vi "콜라자판기(상태머신).vi"() -> ()   [LabVIEW 2014]
uses:
  Status.ctl
panel:
  out "Count Up":i32
  out "그림 링":u16(ring)
  in  "종료":bool
  in  "반환":bool
  in  "구매":bool
  out "투입금액":i32 format="%.0f원"
  in  "동전":T1
  # "콜라자판기"
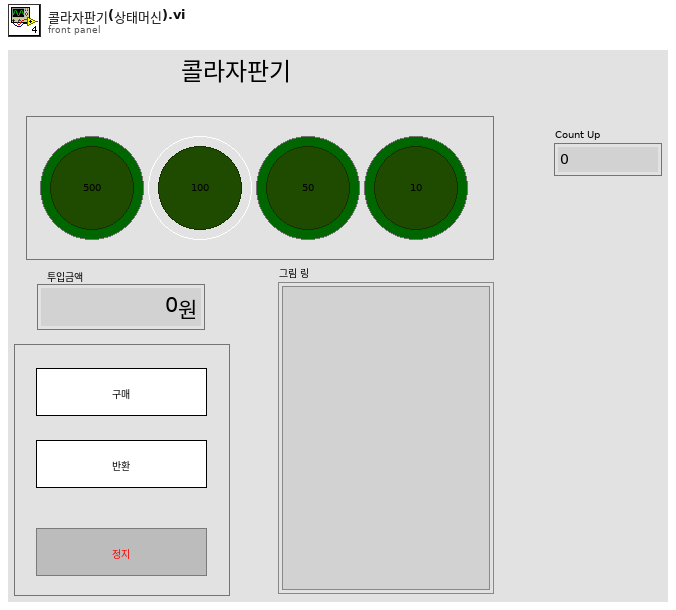
[diagram p1: front panel]
types:
  T1 = cluster{"불리언":bool, "불리언 2":bool, "불리언 3":bool, "불리언 4":bool}
  T2 = typedef "Status.ctl" = enum16{"Idle", "초기화", "종료", "구매", "반환", "1초기다림"}
  T3 = enum8{"Enabled", "Disabled", "Disabled and Grayed Out"}
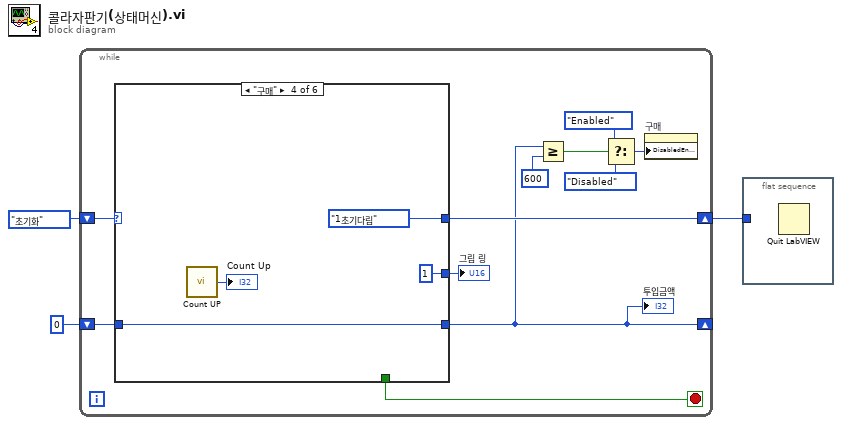
[diagram p0: block diagram]
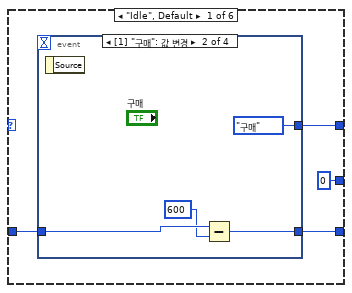
[diagram p2: hidden frame]
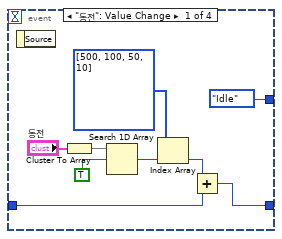
[diagram p3: hidden frame]
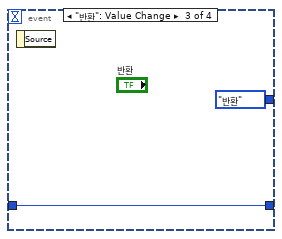
[diagram p4: hidden frame]
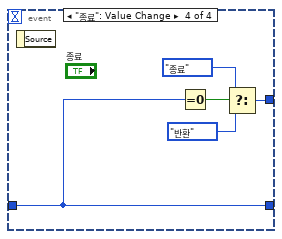
[diagram p5: hidden frame]
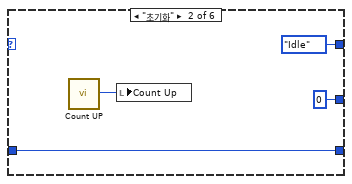
[diagram p6: hidden frame]
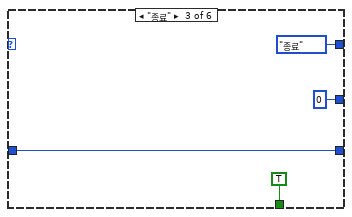
[diagram p7: hidden frame]
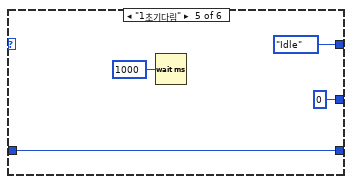
[diagram p8: hidden frame]
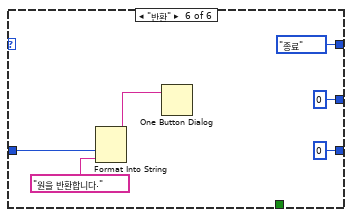
[diagram p9: hidden frame]
diagram:
  n1 = while {
    shift-right: [w13] -> w1
    shift-left: Status."초기화" ("Status") -> [w14]
    shift-right: [w5] -> _
    shift-left: 0 -> [w12]
    stop <- w6 stop-if-true
    n2 = case shown="\"구매\"" w14 {
      tunnel: [w18 Status."Idle" ("Status") Status."종료" ("Status") Status."1초기다림" ("Status") Status."Idle" ("Status") Status."종료" ("Status")] -> w13
      tunnel: w12 -> [w17 w40 w44 w49 w52 w60]
      tunnel: [w16 w40 w44 w49 w52 0] -> w5
      tunnel: [u16 0 u16 0 u16 0 u16 1 u16 0 u16 0] -> w4
      tunnel: [_ _ TRUE _ _ _] -> w6
      frame "Idle", Default {
        n3 = event shown="[1] \"구매\": 값 변경" {
          selector: _ -> [_ _ _ _]
          dyn-events: _ -> [_ _ _ _]
          timeout: _ -> [_ _ _ _]
          tunnel: [Status."Idle" ("Status") Status."구매" ("Status") Status."반환" ("Status") w34] -> w18
          tunnel: w17 -> [w20 w30 w32 w37]
          tunnel: [w19 w29 w32 w37] -> w16
          event "동전": Value Change {
            n4 = event-data() -> ()  [unwired: 1 in, 1 out]
            n5 = Cluster To Array(cluster="동전") -> (array=w25:bool[])
            n6 = Search 1D Array(1D array=w25, element=TRUE) -> (index of element=w23:i32)  [unwired: 1 in]
            n7 = Index Array(array=i32[] [500, 100, 50, 10], index=w23) -> (element=w21:i32)
            n8 = Add(x=w21, y=w20) -> (x+y=w19:i32)
          }
          event "구매": Value Change {
            n9 = event-data() -> ()  [unwired: 1 in, 1 out]
            n10 = Subtract(x=w30, y=600) -> (x-y=w29:i32)
          }
          event "반환": Value Change {
            n11 = event-data() -> ()  [unwired: 1 in, 1 out]
          }
          event "종료": Value Change {
            n12 = event-data() -> ()  [unwired: 1 in, 1 out]
            n13 = Equal To 0?(x=w37) -> (x = 0?=w38:bool)
            n14 = Select(t=Status."종료" ("Status"), s=w38, f=Status."반환" ("Status")) -> (s? t:f=w34:T2)
          }
        }
      }
      frame "초기화" {
        n15 = call "Count UP.vi"() -> ("Count Up"=w39:i32)
        n16 = local write "Count Up"(w39) -> ()
      }
      frame "종료" {
      }
      frame "구매" {
        n17 = call "Count UP.vi"() -> ("Count Up"=→"Count Up":i32)
      }
      frame "1초기다림" {
        n18 = Wait (ms)(milliseconds to wait=u32 1000 ("대기 시간(ms)")) -> ()  [unwired: 1 out]
      }
      frame "반환" {
        n19 = Format Into String(w60, "원을 반환합니다.") -> (resulting string=w58:string)  [unwired: 3 in, 1 out]
        n20 = One Button Dialog(message=w58) -> ()  [unwired: 1 in, 1 out]
      }
    }
    "투입금액" <- w5
    "그림 링" <- w4
    n21 = Greater Or Equal?(x=w5, y=600) -> (x >= y?=w10:bool)
    n22 = Select(t=T3."Enabled" ("비활성화"), s=w10, f=T3."Disabled" ("비활성화")) -> (s? t:f=w7:T3)
    n23 = property on="구매" class="Bool"("DisabledEnum"=w7) -> ()  [unwired: 2 in, 2 out]
  }
  n24 = flat-sequence {
    tunnel: w1 -> [_]
    frame #0 {
      n25 = Quit LabVIEW() -> ()  [unwired: 1 in]
    }
  }
